vi "CSV Data File Parser.vi"(8 "error in":errorcluster, 10 "CSV String":string, 11 "CSV File Path":path) -> (0 "error out":errorcluster, 2 "2-D Array":string[][](table), 3 "Path out":path)   [LabVIEW 2019]
doc: "<b>http://en.wikipedia.org/wiki/Comma-separated_values</b>\n\nReads a CSV formatted text file into a 2D array of strings. The LabVIEW standard Read from Spreadsheet File VI does not support escaped commas or fields that contain CR or LF elements as outlined in RFC 4180\n\nRev 0.2.0 06/08/2011 P. Brooks\n Added feature to replace opening and closing double quotes (0x93 & 0x94) with simple quote (0x22).\n\nRev 0.1.0 05/31/2011 P. Brooks\n Added option to handle strings. If CSV string is NULL (default) then the file in CSV File Path will be parsed instead of CSV string.\n\nRev 0.0.0 05/09/2011 P. Brooks\n Originated."
panel:
  # "http://en.wikipedia.org/wiki/Comma-separated_values"
  # "http://tools.ietf.org/html/rfc4180"
  # "Wikipedia Example Text \n(using opening and closing quotes)"
  # "Year,Make,Model,Description,Price\n1997,Ford,E350, “ac, abs, moon”,3000.00\n1999,Chevy,“Venture ““Extended Edition”””,“”,4900.00\n1999,Chevy,“ Venture ““ Extended Edition, Very Large”””,“”,5000.00\n1996,Jeep,Grand Cherokee,“MUST SELL!\nair, moon roof, loaded”,4799.00"
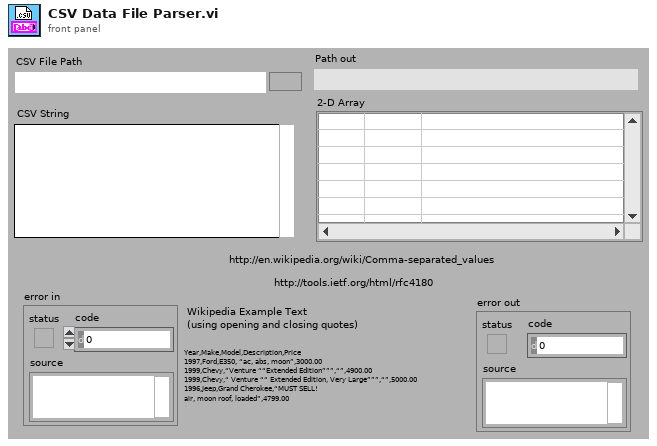
[diagram p1: front panel]
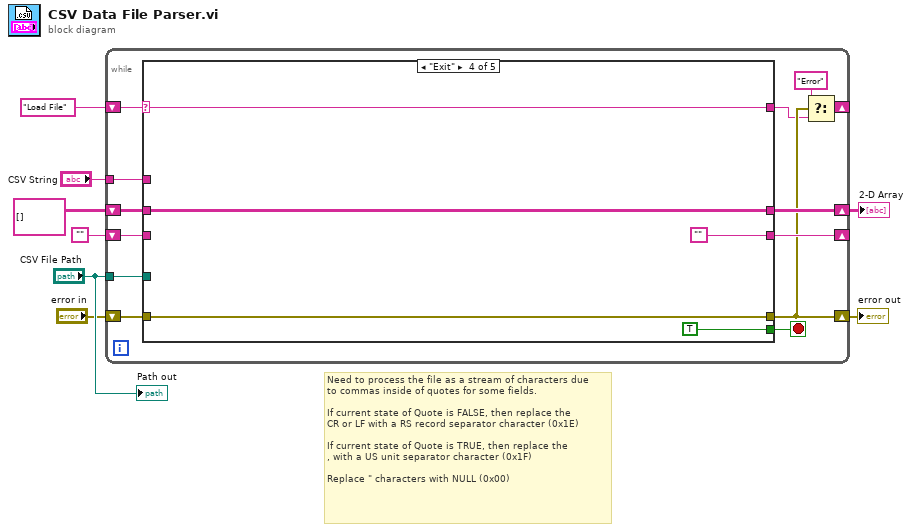
[diagram p0: block diagram]
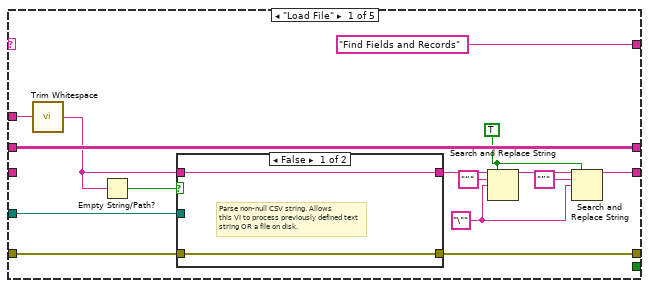
[diagram p2: hidden frame]
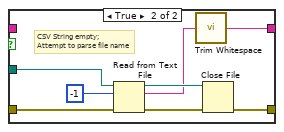
[diagram p3: hidden frame]
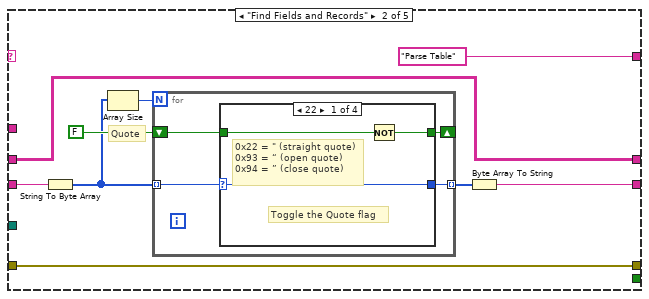
[diagram p4: hidden frame]
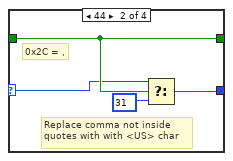
[diagram p5: hidden frame]
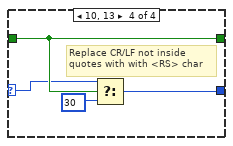
[diagram p7: hidden frame]
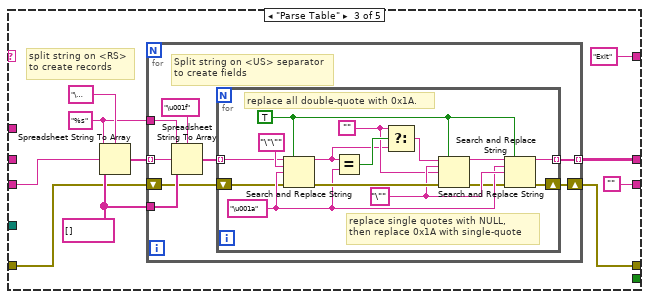
[diagram p8: hidden frame]
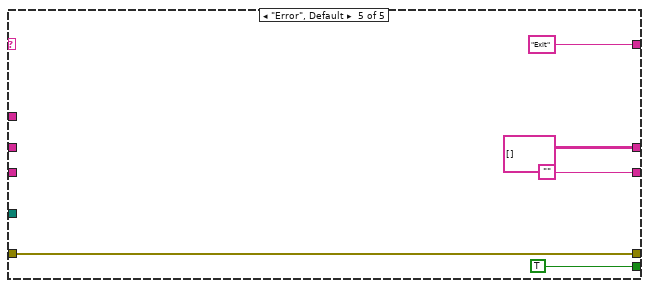
[diagram p9: hidden frame]
diagram:
  # "Need to process the file as a stream of characters due \nto commas inside of quotes for some fields.\n\nIf current state of Quote is FALSE, then replace the\nCR or LF with a RS record separator character (0x1E)\n\nIf current state of Quote is TRUE, then replace the\n, with a US unit separator character (0x1F)\n\nReplace \" characters with NULL (0x00)"
  n1 = while {
    tunnel: "CSV File Path" -> [w20]
    shift-right: [w21] -> _
    shift-left: "" -> [w19]
    shift-right: [w11] -> _
    shift-left: "Load File" -> [w16]
    shift-right: [w18] -> w2
    shift-left: string[][] [] -> [w17]
    shift-right: [w14] -> w3
    shift-left: "error in" -> [w15]
    tunnel: "CSV String" -> [w9]
    stop <- w10 stop-if-true
    n2 = case shown="\"Exit\"" w16 {
      selector: w16 -> [_ _ _ w109 _]
      tunnel: [w25 w50 "" "" ""] -> w21
      tunnel: w20 -> [w32 _ _ _ _]
      tunnel: ["Find Fields and Records" "Parse Table" "Exit" ("t") w109 "Exit" ("t")] -> w13
      tunnel: [_ _ _ TRUE TRUE] -> w10
      tunnel: w19 -> [_ w48 w74 _ _]
      tunnel: [w33 w49 w79 w106 string[][] []] -> w18
      tunnel: w17 -> [w33 w49 _ w106 _]
      tunnel: [w36 w47 w76 w110 w115] -> w14
      tunnel: w15 -> [w35 w47 w73 w110 w115]
      tunnel: w9 -> [w31 _ _ _ _]
      frame "Load File" {
        w22 = TRUE ("replace all? (F)")
        w24 = "\"" ("replace string (\"\")")
        n3 = call <vilib>:"Trim Whitespace.vi"("string"=w31) -> ("trimmed string"=w29:string)  [unwired: 1 in]
        n4 = Empty String/Path?(string/path=w29) -> (empty?=w30:bool)
        n5 = case shown="False" w30 {
          tunnel: [w37 w46] -> w36
          tunnel: w35 -> [w37 w45]
          tunnel: w32 -> [_ w44]
          tunnel: [w38 w39] -> w28
          tunnel: w29 -> [w38 _]
          frame False {
            # "Parse non-null CSV string. Allows\nthis VI to process previously defined text\nstring OR a file on disk."
          }
          frame True {
            # "CSV String empty;\nAttempt to parse file name"
            n6 = Read from Text File(file (use dialog)=w44, count=-1, error in=w45) -> (refnum out=w43:refnum<file>, text=w40:string, error out=w41:errorcluster)  [unwired: 2 out]
            n7 = call <vilib>:"Trim Whitespace.vi"("string"=w40) -> ("trimmed string"=w39:string)  [unwired: 1 in]
            n8 = Close File(refnum=w43, error in=w41) -> (error out=w46:errorcluster)  [unwired: 1 out]
          }
        }
        n9 = Search and Replace String(replace all?=w22, input string=w28, search string="“", replace string=w24) -> (result string=w26:string)  [unwired: 1 in, 6 out]
        n10 = Search and Replace String(replace all?=w22, input string=w26, search string="”", replace string=w24) -> (result string=w25:string)  [unwired: 1 in, 6 out]
      }
      frame "Find Fields and Records" {
        # "Quote"
        n11 = String To Byte Array(string=w48) -> (unsigned byte array=w53:u8[])
        n12 = Array Size(array=w53) -> (size(s)=w54:i32)
        n13 = for {
          N: w54 -> [_]
          tunnel: w53 -> [w56] mode=indexing
          shift-right: [w58] -> _
          shift-left: FALSE -> [w59]
          tunnel: [w57] -> w51 mode=indexing
          n14 = case shown="22" w56 {
            selector: w56 -> [w61 w65 w67 w69]
            tunnel: w59 -> [w60 w66 w68 w72]
            tunnel: [w62 w66 w68 w72] -> w58
            tunnel: [w61 w63 w67 w70] -> w57
            frame 34 {
              # "0x22 = \" (straight quote)\n0x93 = “ (open quote)\n0x94 = ” (close quote)"
              # "Toggle the Quote flag"
              n15 = Not(x=w60) -> (.not. x?=w62:bool)
            }
            frame 44 {
              # "0x2C = ,"
              # "Replace comma not inside \nquotes with with <US> char"
              n16 = Select(t=w65, s=w66, f=u8 31) -> (s? t:f=w63:u8)
            }
            frame 0, Default {
            }
            frame 10, 13 {
              # "Replace CR/LF not inside \nquotes with with <RS> char"
              n17 = Select(t=w69, s=w72, f=u8 30) -> (s? t:f=w70:u8)
            }
          }
        }
        n18 = Byte Array To String(unsigned byte array=w51) -> (string=w50:string)
      }
      frame "Parse Table" {
        w82 = string[] []
        w77 = "%s" ("format string")
        # "split string on <RS>\nto create records"
        n19 = Spreadsheet String To Array(delimiter (Tab)="\u001e", format string=w77, spreadsheet string=w74, array type (2D Dbl)=w82) -> (array=w81:string[])
        n20 = for {
          tunnel: w81 -> [w90] mode=indexing
          tunnel: w82 -> [w87]
          tunnel: [w86] -> w79 mode=indexing
          tunnel: w77 -> [w85]
          shift-right: [w83] -> w76
          shift-left: w73 -> [w84]
          # "Split string on <US> separator\nto create fields"
          n21 = Spreadsheet String To Array(delimiter (Tab)="\u001f", format string=w85, spreadsheet string=w90, array type (2D Dbl)=w87) -> (array=w88:string[])
          n22 = for {
            tunnel: w88 -> [w91] mode=indexing
            tunnel: [w92] -> w86 mode=indexing
            shift-right: [w93] -> w83
            shift-left: w84 -> [w95]
            w98 = ""
            w101 = "\"" ("input string")
            w102 = TRUE ("replace all? (F)")
            w100 = "\u001a" ("replace string (\"\")")
            # "replace single quotes with NULL,\nthen replace 0x1A with single-quote"
            # "replace all double-quote with 0x1A."
            n23 = Search and Replace String(replace all?=w102, input string=w91, search string="\"\"", replace string=w100, error in=w95) -> (result string=w97:string, error out=w104:errorcluster)  [unwired: 5 out]
            n24 = Equal?(x=w97, y=w100) -> (x = y?=w99:bool)
            n25 = Select(t=w98, s=w99, f=w97) -> (s? t:f=w96:string)
            n26 = Search and Replace String(replace all?=w102, input string=w96, search string=w101, replace string=w98, error in=w104) -> (result string=w103:string, error out=w94:errorcluster)  [unwired: 5 out]
            n27 = Search and Replace String(replace all?=w102, input string=w103, search string=w100, replace string=w101, error in=w94) -> (result string=w92:string, error out=w93:errorcluster)  [unwired: 1 in, 4 out]
          }
        }
      }
      frame "Exit" {
      }
      frame "Error", Default {
      }
    }
    n28 = Select(t="Error", s=w14, f=w13) -> (s? t:f=w11:string)
  }
  "error out" <- w3
  "2-D Array" <- w2
  "Path out" <- "CSV File Path"
